vi "WebAPI_Excel.vi"(8 "error in (no error)":errorcluster) -> (0 "error out":errorcluster)   [LabVIEW 2014]
uses:
  <vilib>/httpClient/POSTBuffer.vi
  <vilib>/Utility/file.llb/Write To Spreadsheet File (string).vi
  <vilib>/httpClient/LabVIEWHTTPClient.lvlib
panel:
  out "length":i32
  out "CSV_out":string[][](array[string])
  out "value":T1(array[cluster])
  in  "Array":T1(array[cluster])
  out "body":string
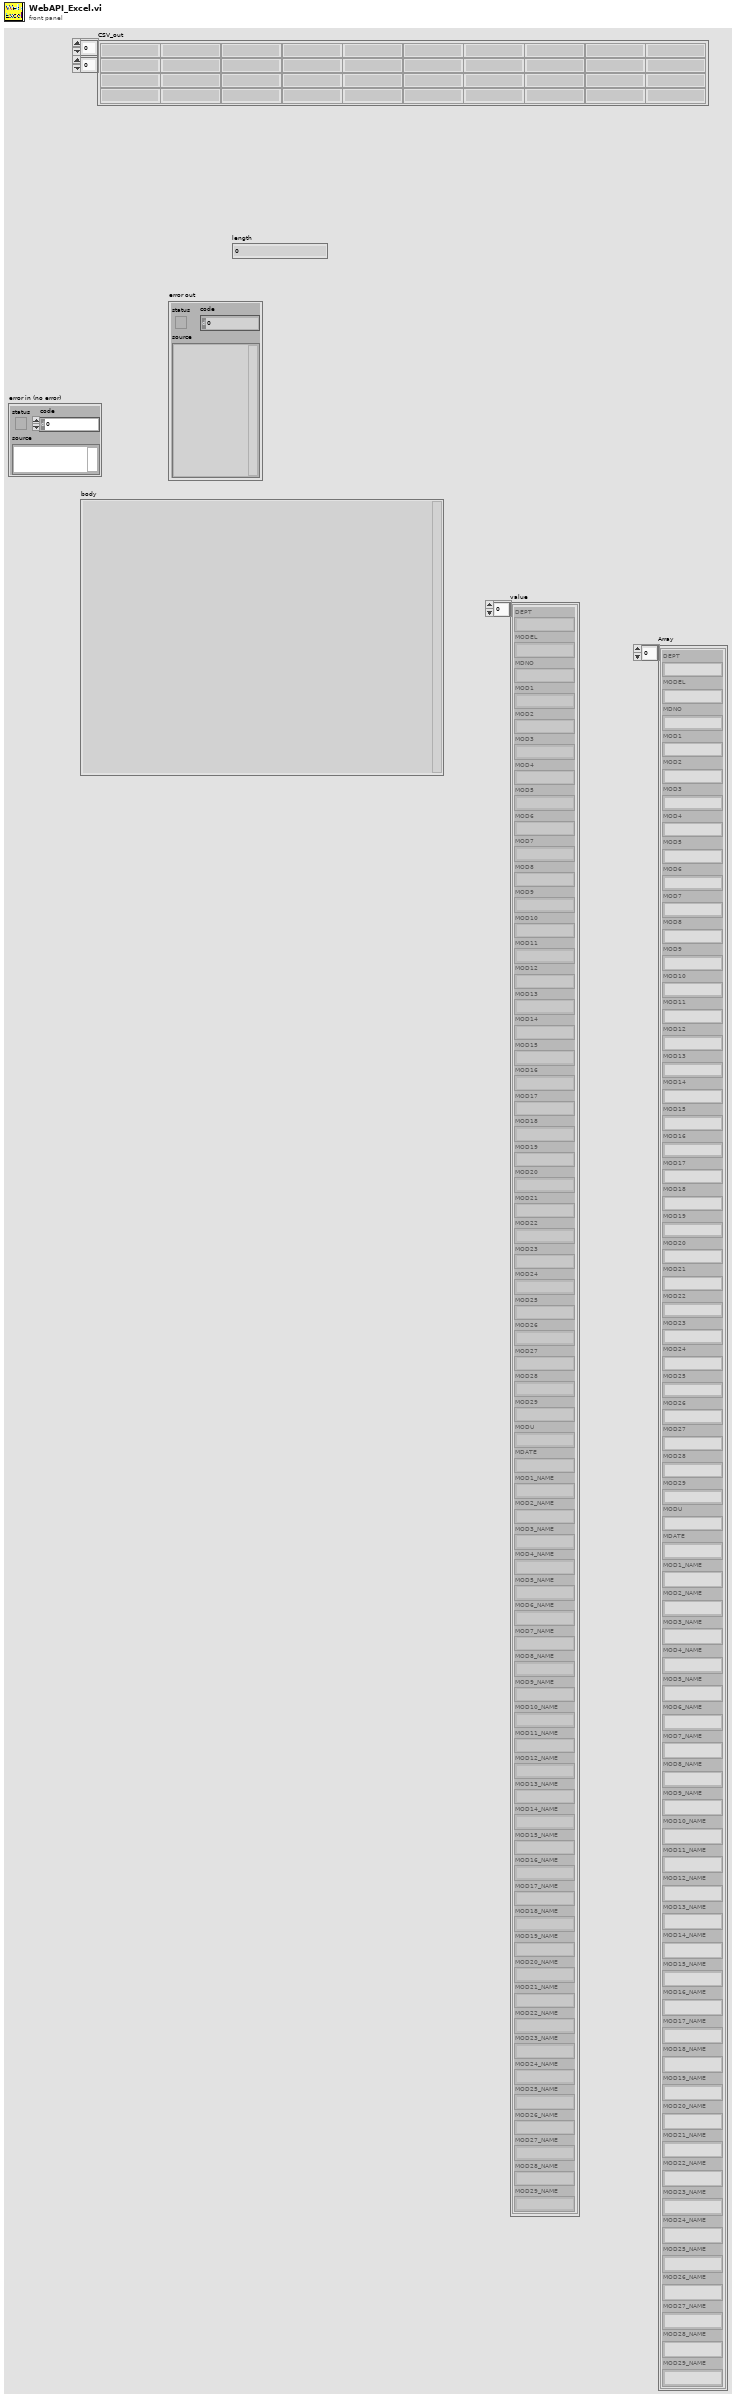
[diagram p1: front panel]
types:
  T1 = cluster{"DEPT":string, "MODEL":string, "MDNO":string, "MOD1":string, "MOD2":string, "MOD3":string, "MOD4":string, "MOD5":string, "MOD6":string, "MOD7":string, "MOD8":string, "MOD9":string, "MOD10":string, "MOD11":string, "MOD12":string, "MOD13":string, "MOD14":string, "MOD15":string, "MOD16":string, "MOD17":string, "MOD18":string, "MOD19":string, "MOD20":string, "MOD21":string, "MOD22":string, "MOD23":string, "MOD24":string, "MOD25":string, "MOD26":string, "MOD27":string, "MOD28":string, "MOD29":string, "MODU":string, "MDATE":string, "MOD1_NAME":string, "MOD2_NAME":string, "MOD3_NAME":string, "MOD4_NAME":string, "MOD5_NAME":string, "MOD6_NAME":string, "MOD7_NAME":string, "MOD8_NAME":string, "MOD9_NAME":string, "MOD10_NAME":string, "MOD11_NAME":string, "MOD12_NAME":string, "MOD13_NAME":string, "MOD14_NAME":string, "MOD15_NAME":string, "MOD16_NAME":string, "MOD17_NAME":string, "MOD18_NAME":string, "MOD19_NAME":string, "MOD20_NAME":string, "MOD21_NAME":string, "MOD22_NAME":string, "MOD23_NAME":string, "MOD24_NAME":string, "MOD25_NAME":string, "MOD26_NAME":string, "MOD27_NAME":string, "MOD28_NAME":string, "MOD29_NAME":string}[]
  T2 = typedef "LabVIEWHTTPClient.lvlib/ClientHandle.ctl" = refnum<k1>
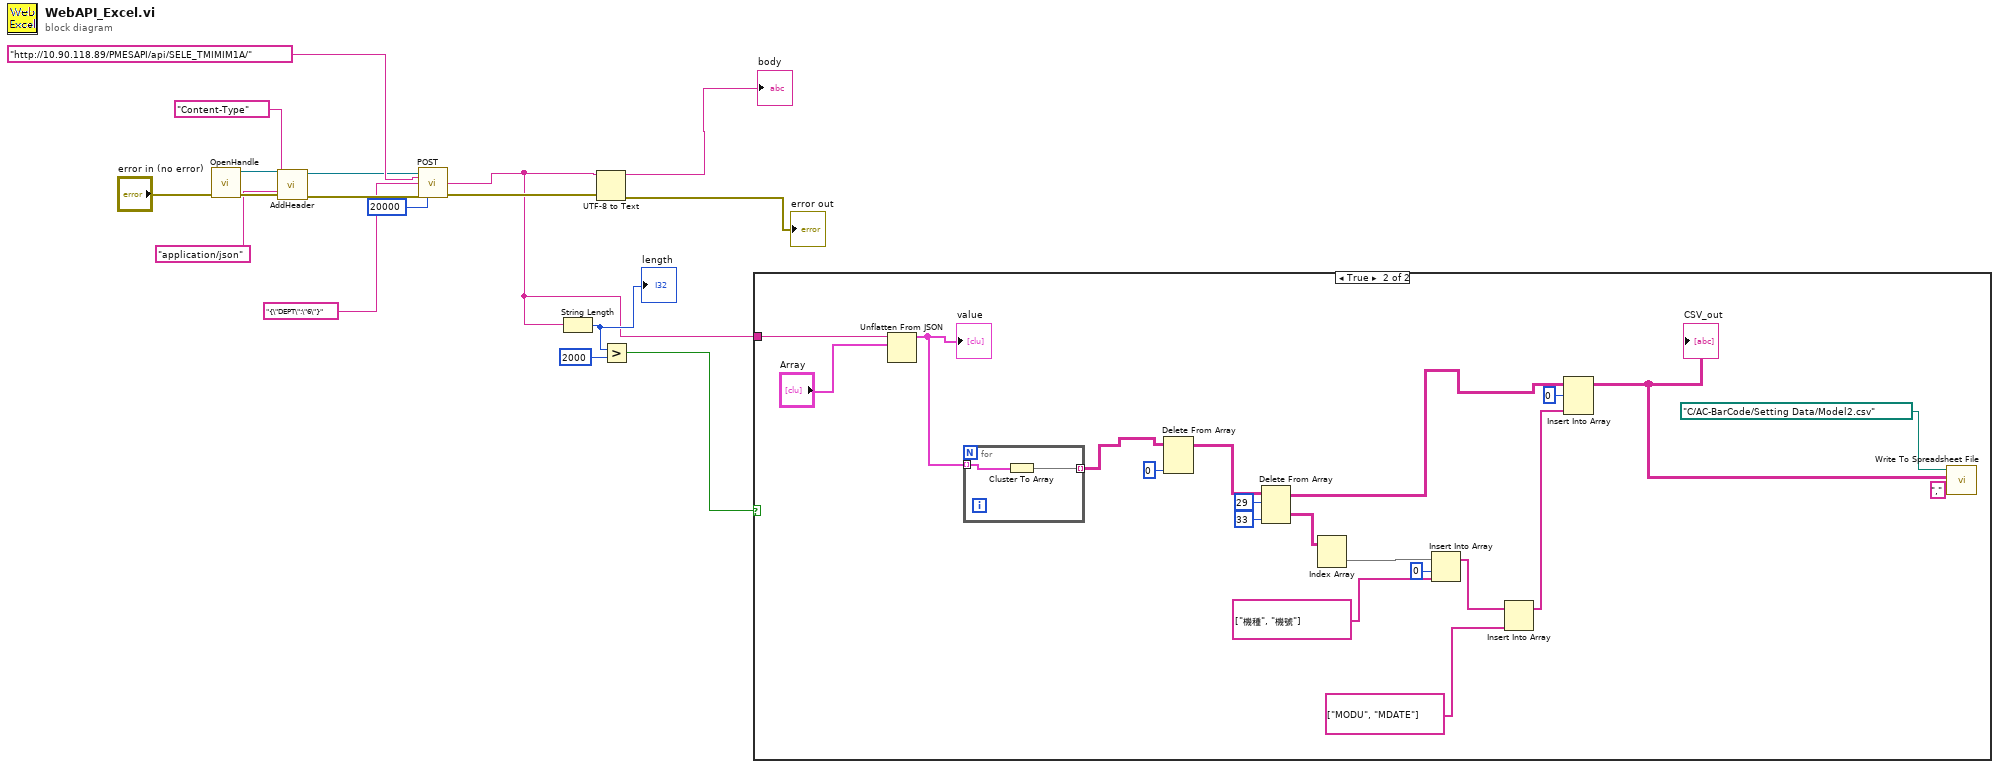
[diagram p0: block diagram]
diagram:
  n1 = call <vilib>:"OpenHandle.vi"("error in (no error)"="error in (no error)") -> ("client handle out"=w17:T2, "error out"=w16:errorcluster)  [unwired: 13 in]
  n2 = call <vilib>:"AddHeader.vi"("client handle"=w17, "header"="Content-Type", "value"="application/json", "error in (no error)"=w16) -> ("client handle out"=w12:T2, "error out"=w11:errorcluster)  [unwired: 10 in]
  n3 = call-poly <vilib>:"POST.vi"("client handle"=w12, "url"="http://10.90.118.89/PMESAPI/api/SELE_TMIMIM1A/", "buffer"="{\"DEPT\":\"6\"}", "error in (no error)"=w11, "timeout (10000)"=20000) -> ("body"=w2:string, "error out"=w8:errorcluster)  [unwired: 7 in, 2 out]
  n4 = String Length(string=w2) -> (length=w5:i32)
  "length" <- w5
  n5 = UTF-8 to Text(8:w8, 11:w2) -> (0:→"error out":errorcluster, 3:→"body":string)  [unwired: 1 in]
  n6 = Greater?(x=w5, y=2000) -> (0:w3:bool)
  n7 = case shown="True" w3 {
    tunnel: w2 -> [_ w18]
    frame False {
    }
    frame True {
      n8 = Unflatten From JSON(JSON string=w18, type and defaults="Array") -> (value=w36:T1)  [unwired: 5 in, 1 out]
      "value" <- w36
      n9 = for {
        tunnel: w36 -> [w39] mode=indexing
        tunnel: [w38] -> w35 mode=indexing
        n10 = Cluster To Array(cluster=w39) -> (array=w38:string[])
      }
      n11 = Delete From Array(array=w35, index (col)=0 ("disabled index (col)")) -> (array with subset deleted=w33:string[][])  [unwired: 2 in, 1 out]
      n12 = Delete From Array(array=w33, length=29, index (col)=33 ("disabled index (col)")) -> (deleted portion=w30:string[][], array with subset deleted=w24:string[][])  [unwired: 1 in]
      n13 = Index Array(array=w30) -> (element=w29:string[])  [unwired: 2 in]
      n14 = Insert Into Array "Insert Into Array"(array=w29, index=0, new element=string[] ["機種", "機號"]) -> (w26:string[])
      n15 = Insert Into Array "Insert Into Array"(array=w26, new element=string[] ["MODU", "MDATE"]) -> (w23:string[])  [unwired: 1 in]
      n16 = Insert Into Array(array=w24, index (row)=0, new element=w23) -> (w20:string[][])  [unwired: 1 in]
      "CSV_out" <- w20
      n17 = call-poly <vilib>:"Write To Spreadsheet File.vi"("delimiter (\\t)"="," ("delimiter (\\t)"), "2D data"=w20, "file path (dialog if empty)"=path "C:/AC-BarCode/Setting Data/Model2.csv") -> ()  [unwired: 5 in, 1 out]
    }
  }
